vi "Set Board Properties.vi"(8 "error in":errorcluster, 10 "board setup":T2 {"portConfig" items=["FDX_SINGLE", "FDX_REDUNDANT"]; "portSpeed" items=["FDX_100MBIT", "FDX_10MBIT", "FDX_AUTO_100MBIT", "FDX_AUTO_10MBIT", "FDX_AUTO_ERROR", "FDX_1000MBIT"]}, 11 "custom device ref in":T1 format="%.0x") -> (0 "error out":errorcluster, 2 "redundant?":bool, 3 "custom device ref out":T1 format="%.0x")   [LabVIEW 2020, in "AIM ARINC 664 Scripting.lvlib"]
doc: "Set board properties as board ID, Port Speed and Port Configuration."
uses:
  AIM ARINC 664 Scripting.lvlib
  Import/_typedefs/board_setup.ctl
  <vilib>/NI VeriStand/Custom Device API/Custom Device Item Ref.ctl
  Import/AIM ARINC 664 Import.lvlib
  <vilib>/NI VeriStand/Custom Device API/Custom Device API.lvlib
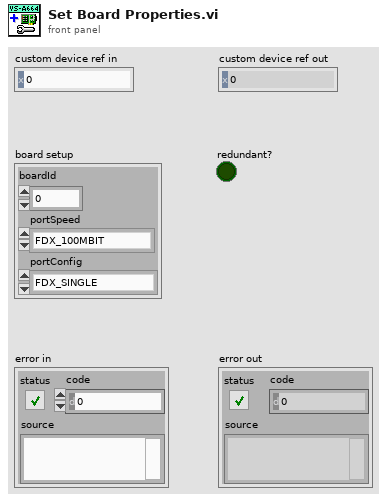
[diagram p1: front panel]
types:
  T1 = typedef "Custom Device API.lvlib/Custom Device Item Ref.ctl" = u64
  T2 = typedef "AIM ARINC 664 Import.lvlib/board_setup.ctl" = cluster{"boardId":u32, "portSpeed":u32, "portConfig":u32}
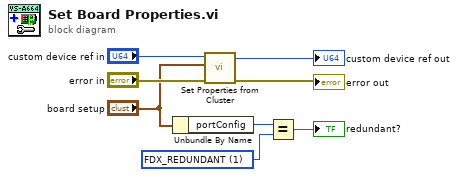
[diagram p0: block diagram]
diagram:
  w6 = u32 1 items=["FDX_SINGLE", "FDX_REDUNDANT"] ("portConfig")
  n1 = Unbundle By Name("board setup") -> ("portConfig"=w8:u32)
  n2 = call "Set Properties from Cluster.vi"("error in"="error in", "Variant Cluster"="board setup", "item ref in"="custom device ref in") -> ("error out"=→"error out":errorcluster, "item ref out"=→"custom device ref out":T1)  [unwired: 7 in]
  n3 = Equal?(x=w8, y=w6) -> (x = y?=→"redundant?":bool)
